vi "Solar Cell Parameters Measuring.vi"() -> ()   [LabVIEW 2019]
uses:
  <vilib>/Analysis/baseanly.llb/Mean (DBL).vi
  <vilib>/DAQmx/create/channels.llb/DAQmx Create Channel (AI-Voltage-Basic).vi
  <vilib>/DAQmx/configure/timing.llb/DAQmx Timing (Sample Clock).vi
  <vilib>/DAQmx/create/channels.llb/DAQmx Create Channel (AO-Voltage-Basic).vi
  <vilib>/DAQmx/miscellaneous.llb/DAQmx Fill In Error Info.vi
  <vilib>/express/express shared/transition.llb/Dynamic To Waveform Array.vi
  <vilib>/express/express signal manip/GetorSetDDTAttributes/Set DDT Attributes/SetT0.vi
  <vilib>/express/express shared/transition.llb/Waveform Array To Dynamic.vi
  <vilib>/express/express signal manip/GetorSetDDTAttributes/Set DDT Attributes/Set DDT Properties.xnode
  <vilib>/DAQmx/read.llb/DAQmx Read (Analog 2D DBL NChan NSamp).vi
  <vilib>/DAQmx/write.llb/DAQmx Write (Analog 1D DBL NChan 1Samp).vi
  <vilib>/DAQmx/read.llb/DAQmx Read (Analog DBL 1Chan 1Samp).vi
  <vilib>/DAQmx/create/channels.llb/DAQmx Create Channel (AI-Temperature-Thermocouple).vi
  <vilib>/Analysis/NI_AALBase.lvlib
  <vilib>/Analysis/NI_AALPro.lvlib
panel:
  in  "Tab Control":enum32{"Parameters", "I-V Curve", "Calibration"}(tab)
  in  "GAIN x":u16(ring)=1000 items=["100"=100, "1000"=1000, "10"=10, "1"=1]
  out "Rseries":dbl format="%#.3g"
  out "Rshunt":dbl format="%#.3g"
  out "Progress":u8(slide)=100 scale=0.0..100.0
  in  "Save File":bool
  in  "S (cm2)":dbl=0.0324
  in  "P  (mW/cm2)":dbl=100.0
  in  "Points":dbl=400.0
  out "Voc  ( V )":dbl format="%#_2g"
  out "Isc  (  mA  )":dbl format="%#_3g"
  out "Imp (mA)":dbl format="%#_3g"
  out "Vmp  (V)":dbl format="%#_2g"
  out "Max  Power  ( mW )":dbl format="%#_2g"
  out "u (%)":dbl format="%#_2g"
  out "FF":dbl format="%#_2g"
  out "Current and Power vs. Voltage":cluster{"voltage":dbl[], "current":dbl[]}[](graph)
  out "Rs":dbl format="%#_3g"
  out "Trmerature Celsius":dbl format="%0.2f"
  in  "File Name":string="Name"
  in  "Grid":enum32{"Radio Selection 1", "Radio Selection 2"}(radio)=enum."Radio Selection 2"
  out "Current (Amps) vs Voltage (Volts)":cluster{"Array":dbl[], "Array":dbl[]}[](graph)
  in  "percentage":sgl=0.075
  in  "100x":dbl=0.00220747 format="%#_13g"
  in  "1000x":dbl=0.01825644 format="%#_13g"
  in  "10x":dbl=0.00069563 format="%#_13g"
  in  "1x":dbl=0.00053122 format="%#_13g"
  out "Gain Coepicient":dbl format="%0.8f"
  out "task out 2":refnum<k21>
  out "task out":refnum<k21>
  # "%"
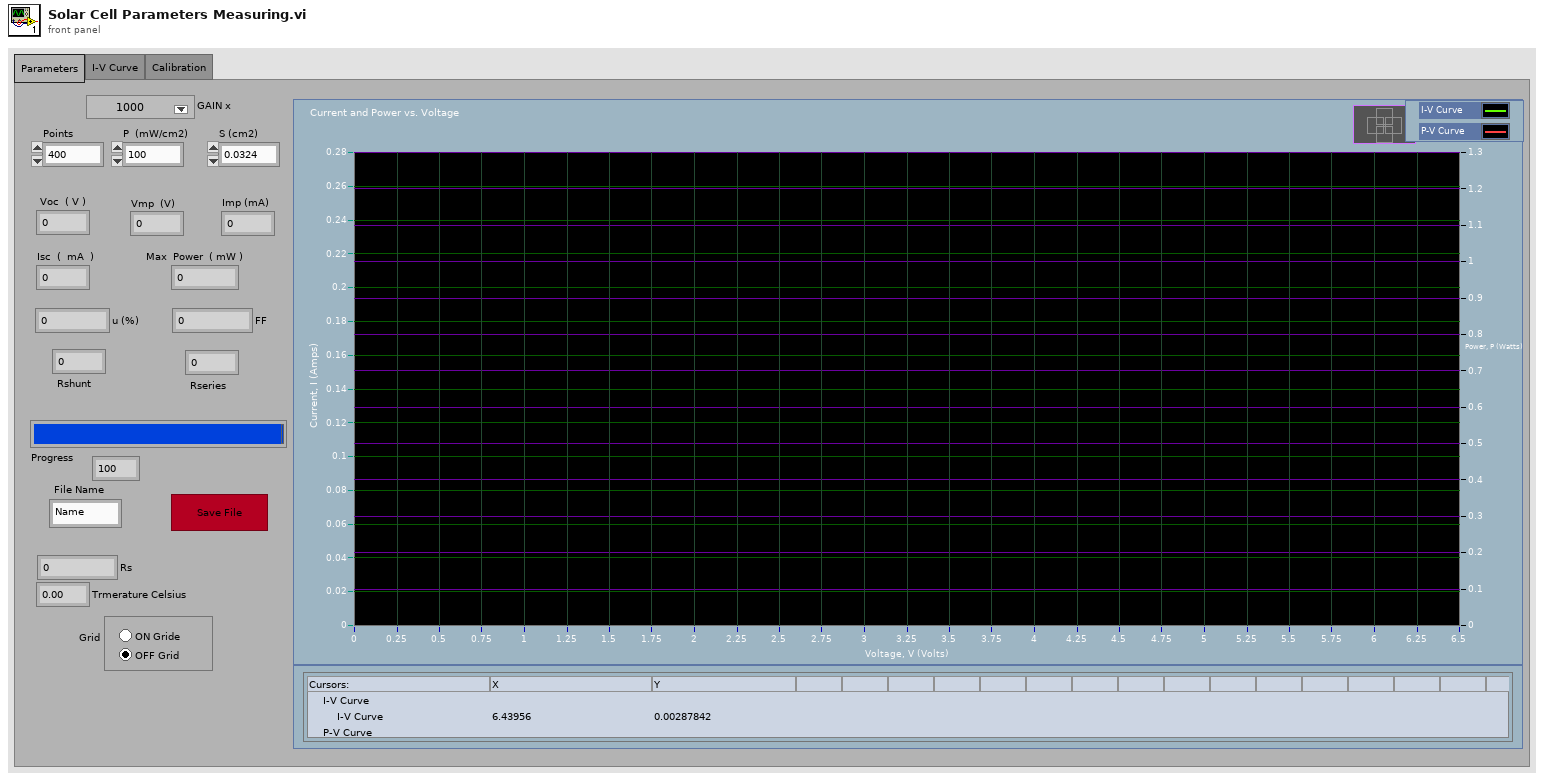
[diagram p1: front panel]
types:
  T1 = typedef "imagedata.ctl" = cluster{"image type":i32, "image depth":i32, "image":u8[], "mask":u8[], "colors":u32[], "Rectangle":cluster{"left":i16, "top":i16, "right":i16, "bottom":i16}}
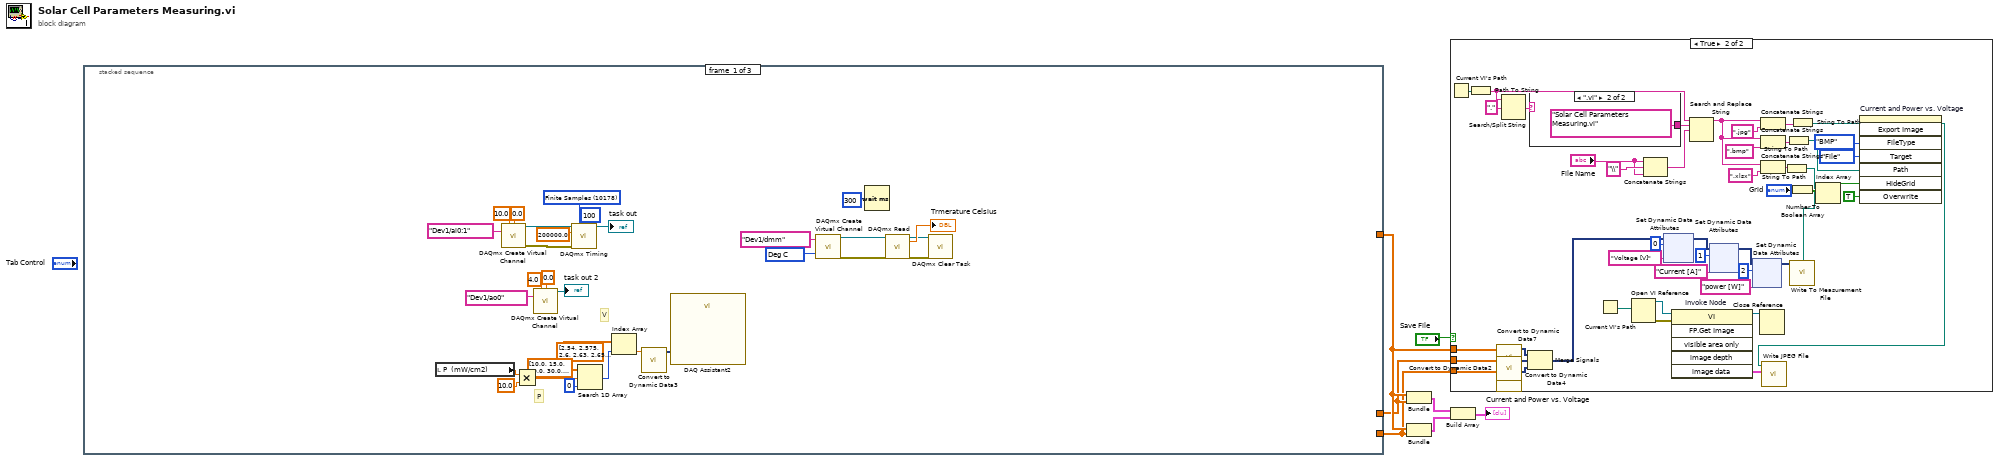
[diagram p0: block diagram]
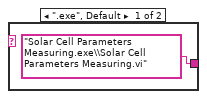
[diagram p3: hidden frame]
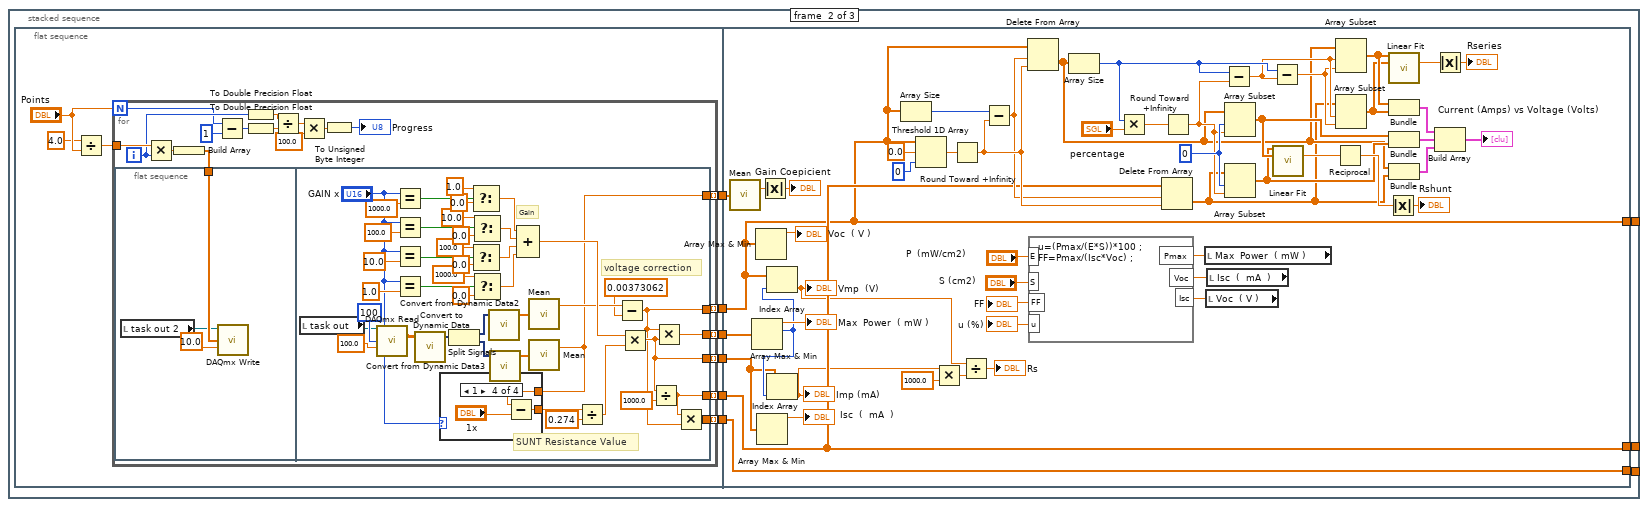
[diagram p4: hidden frame]
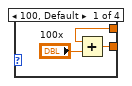
[diagram p5: hidden frame]
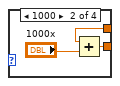
[diagram p6: hidden frame]
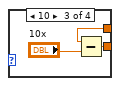
[diagram p7: hidden frame]
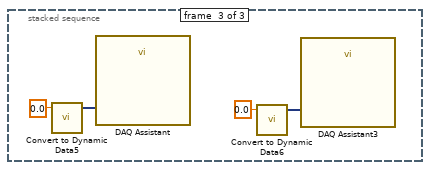
[diagram p8: hidden frame]
diagram:
  n1 = stacked-sequence {
    tunnel: [_ w43 _] -> w3
    tunnel: [_ w40 _] -> w2
    tunnel: [_ w39 _] -> w1
    frame #0 {
      w20 = 10143 items=["Deg C"=10143, "Deg F"=10144, "Kelvins"=10325, "Deg R"=10145, "From Custom Scale"=10065] ("units")
      w26 = 10178 items=["Finite Samples"=10178, "Continuous Samples"=10123, "Hardware Timed Single Point"=12522] ("sample mode")
      # "P"
      # "V"
      n2 = local read "P  (mW/cm2)"() -> (w15:dbl)
      n3 = call-poly <vilib>:"DAQmx Create Virtual Channel.vi"("maximum value"=10.0, "minimum value"=0.0, "physical channels"=tag "Dev1/ai0:1") -> ("task out"=w29:refnum<k21>, "error out"=w28:errorcluster)  [unwired: 11 in]
      n4 = Multiply(x=w15, y=10.0) -> (x*y=w9:dbl)
      n5 = call-poly <vilib>:"DAQmx Create Virtual Channel.vi"("maximum value"=4.0, "minimum value"=0.0, "physical channels"=tag "Dev1/ao0") -> ("task out"=→"task out 2":refnum<k21>)  [unwired: 11 in, 1 out]
      n6 = call-poly <vilib>:"DAQmx Timing.vi"("task/channels in"=w29, "sample mode"=w26, "samples per channel"=100, "rate"=200000.0, "error in"=w28) -> ("task out"=→"task out":refnum<k21>)  [unwired: 9 in, 1 out]
      n7 = Search 1D Array(1D array=dbl[] [10.0, 15.0, 20.0, 30.0, 40.0, 50.0, 60.0, 70.0, 80.0, 90.0, 100.0, 120.0, 140.0, 160.0, 180.0, 200.0, 220.0, 240.0, 260.0, 280.0, 300.0, 350.0, 400.0, 450.0, 500.0, 550.0, 600.0, 650.0, 700.0, 750.0, 800.0, 850.0, 900.0, 950.0, 1000.0] ("P"), element=w9, start index (0)=0) -> (index of element=w10:i32)
      n8 = Index Array(array=dbl[] [2.54, 2.575, 2.6, 2.63, 2.653, 2.672, 2.688, 2.7, 2.71, 2.719, 2.728, 2.74, 2.7525, 2.7627, 2.771, 2.779, 2.784, 2.7895, 2.792, 2.7976, 2.8011, 2.81, 2.817, 2.8238, 2.8295, 2.8301, 2.8315, 2.8325, 2.831, 2.833, 2.835, 2.836, 2.838, 2.84, 2.86] ("V"), index=w10) -> (element=w8:dbl)
      n9 = call "Convert to Dynamic Data3"("Double"=w8) -> ("Dynamic Data Type"=w24:dynamicdata)  [unwired: 3 in]
      n10 = call "DAQ Assistant2"("data"=w24) -> ()  [unwired: 17 in, 2 out]
      n11 = call-poly <vilib>:"DAQmx Create Virtual Channel.vi"("physical channels"=tag "Dev1/dmm", "units"=w20) -> ("task out"=w22:refnum<k21>, "error out"=w19:errorcluster)  [unwired: 12 in]
      n12 = Wait (ms)(milliseconds to wait=u32 300) -> ()  [unwired: 1 out]
      n13 = call-poly <vilib>:"DAQmx Read.vi"("task/channels in"=w22, "error in"=w19) -> ("task out"=w17:refnum<k21>, "data"=→"Trmerature Celsius":dbl, "error out"=w16:errorcluster)  [unwired: 11 in]
      n14 = call <vilib>:"DAQmx Clear Task.vi"("task in"=w17, "error in"=w16) -> ()  [unwired: 13 in, 1 out]
    }
    frame #1 {
      n15 = flat-sequence {
        tunnel: [w52] -> w46
        tunnel: [w51] -> w45
        tunnel: [w50] -> w44
        tunnel: [w49] -> w42
        tunnel: [w48] -> w41
        tunnel: [w47] -> w38
        tunnel: w46 -> [w144]
        tunnel: w45 -> [w136]
        tunnel: w44 -> [w180]
        tunnel: [w144] -> w43
        tunnel: w42 -> [w145]
        tunnel: [w145] -> w40
        tunnel: w41 -> [w142]
        tunnel: [w142] -> w39
        tunnel: w38 -> [w135]
        frame #0 {
          n16 = Divide(x=4.0, y="Points") -> (x/y=w55:dbl)
          n17 = for {
            N: "Points" -> [w62]
            tunnel: w55 -> [w72]
            tunnel: [w61] -> w50 mode=indexing
            tunnel: [w59] -> w52 mode=indexing
            tunnel: [w60] -> w51 mode=indexing
            tunnel: [w58] -> w49 mode=indexing
            tunnel: [w57] -> w48 mode=indexing
            tunnel: [w56] -> w47 mode=indexing
            i -> [w63]
            n18 = flat-sequence {
              tunnel: w74 -> [w77]
              tunnel: [w109] -> w61
              tunnel: [w108] -> w60
              tunnel: [w81] -> w59
              tunnel: [w106] -> w58
              tunnel: [w105] -> w57
              tunnel: [w79] -> w56
              frame #0 {
                n19 = local read "task out 2"() -> (w75:refnum<k21>)
                n20 = call-poly <vilib>:"DAQmx Write.vi"("task/channels in"=w75, "data"=w77, "timeout"=10.0) -> ()  [unwired: 10 in, 3 out]
              }
              frame #1 {
                # "voltage correction"
                # "SUNT Resistance Value"
                # "Gain"
                n21 = local read "task out"() -> (w110:refnum<k21>)
                n22 = call-poly <vilib>:"DAQmx Read.vi"("task/channels in"=w110, "number of samples per channel"=100, "timeout"=100.0) -> ("data"=w115:dbl[][])  [unwired: 10 in, 2 out]
                n23 = Equal?(x="GAIN x", y=1000.0) -> (x = y?=w89:bool)
                n24 = Equal?(x="GAIN x", y=100.0) -> (x = y?=w90:bool)
                n25 = Equal?(x="GAIN x", y=10.0) -> (x = y?=w91:bool)
                n26 = Equal?(x="GAIN x", y=1.0) -> (x = y?=w92:bool)
                n27 = call "Convert to Dynamic Data"("2D Array"=w115) -> ("Dynamic Data Type"=w114:dynamicdata)  [unwired: 3 in]
                n28 = Split Signals(w114) -> (w113:dynamicdata, w112:dynamicdata)  [unwired: 2 in]
                n29 = Select(t=1.0 ("Double"), s=w89, f=0.0) -> (s? t:f=w97:dbl)
                n30 = Select(t=100.0 ("Double"), s=w91, f=0.0) -> (s? t:f=w99:dbl)
                n31 = Select(t=10.0 ("Double"), s=w90, f=0.0) -> (s? t:f=w98:dbl)
                n32 = Select(t=1000.0 ("Double"), s=w92, f=0.0) -> (s? t:f=w100:dbl)
                n33 = call "Convert from Dynamic Data2"("Dynamic Data Type"=w113) -> ("Array"=w118:dbl[])  [unwired: 3 in]
                n34 = call "Convert from Dynamic Data3"("Dynamic Data Type"=w112) -> ("Array"=w119:dbl[])  [unwired: 3 in]
                n35 = Compound Arithmetic op=ADD(w97, w98, w99, w100) -> (w84:dbl)
                n36 = call-poly <vilib>:"Mean.vi"("X"=w118) -> ("mean"=w82:dbl)  [unwired: 1 out]
                n37 = call-poly <vilib>:"Mean.vi"("X"=w119) -> ("mean"=w79:dbl)  [unwired: 1 out]
                n38 = case shown="1" "GAIN x" {
                  tunnel: [w121 w126 w129 w131] -> w78
                  tunnel: w79 -> [w122 w124 w128 w132]
                  frame 100, Default {
                    n39 = Add(x=w122, y="100x") -> (x+y=w121:dbl)
                  }
                  frame 1000 {
                    n40 = Add(x=w124, y="1000x") -> (x+y=w126:dbl)
                  }
                  frame 10 {
                    n41 = Subtract(x=w128, y="10x") -> (x-y=w129:dbl)
                  }
                  frame 1 {
                    n42 = Subtract(x=w132, y="1x") -> (x-y=w131:dbl)
                  }
                }
                n43 = Divide(x=w78, y=0.274) -> (x/y=w116:dbl)
                n44 = Subtract(x=w82, y=0.00373062) -> (x-y=w81:dbl)
                n45 = Multiply(x=w84, y=w116) -> (x*y=w108:dbl)
                n46 = Divide(x=w108, y=1000.0) -> (x/y=w106:dbl)
                n47 = Multiply(x=w81, y=w108) -> (x*y=w109:dbl)
                n48 = Multiply(x=w106, y=w81) -> (x*y=w105:dbl)
              }
            }
            n49 = Multiply(x=w72, y=w63) -> (x*y=w73:dbl)
            n50 = Build Array(w73) -> (w74:dbl[])
            n51 = Subtract(x=w62, y=1) -> (x-y=w65:i32)
            n52 = To Double Precision Float(number=w63) -> (double precision float=w66:dbl)
            n53 = To Double Precision Float(number=w65) -> (double precision float=w68:dbl)
            n54 = Divide(x=w66, y=w68) -> (x/y=w70:dbl)
            n55 = Multiply(x=w70, y=100.0) -> (x*y=w67:dbl)
            n56 = To Unsigned Byte Integer(number=w67) -> (unsigned 8bit integer=→"Progress":u8)
          }
        }
        frame #1 {
          w158 = 0 ("index")
          n57 = call-poly <vilib>:"Mean.vi"("X"=w135) -> ("mean"=w134:dbl)  [unwired: 1 out]
          n58 = Array Max & Min(array=w180) -> (max value=→"Max  Power  ( mW )":dbl, max index (indices)=w181:i32)  [unwired: 2 out]
          n59 = Array Max & Min(array=w144) -> (max value=→"Voc  ( V )":dbl)  [unwired: 3 out]
          n60 = Array Max & Min(array=w136) -> (max value=→"Isc  (  mA  )":dbl)  [unwired: 3 out]
          n61 = Absolute Value(x=w134) -> (abs(x)=→"Gain Coepicient":dbl)
          n62 = Index Array(array=w144, index=w181) -> (element=w137:dbl)
          "Vmp  (V)" <- w137
          n63 = Index Array(array=w136, index=w181) -> (element=w139:dbl)
          "Imp (mA)" <- w139
          n64 = Array Size(array=w144) -> (size(s)=w157:i32)
          n65 = Threshold 1D Array(1:0 ("start index (0)"), 2:0.0 ("threshold y"), 3:w144) -> (0:w170:dbl)
          n66 = Multiply(x=w139, y=1000.0) -> (x*y=w140:dbl)
          n67 = Round Toward +Infinity(x=w170) -> (ceil(x): smallest int >= x=w169:dbl)
          n68 = Divide(x=w137, y=w140) -> (x/y=→"Rs":dbl)
          n69 = Subtract(x=w157, y=w169) -> (x-y=w168:dbl)
          n70 = Delete From Array(array=w144, length=w168, index=w169) -> (deleted portion=w152:dbl[])  [unwired: 1 out]
          n71 = Array Size(array=w152) -> (size(s)=w155:i32)
          n72 = Multiply(x=w155, y="percentage") -> (x*y=w163:sgl)
          n73 = Delete From Array(array=w145, length=w168, index=w169) -> (deleted portion=w151:dbl[])  [unwired: 1 out]
          n74 = Round Toward +Infinity(x=w163) -> (ceil(x): smallest int >= x=w156:sgl)
          n75 = local read "Max  Power  ( mW )"() -> (w177:dbl)
          n76 = local read "Voc  ( V )"() -> (w179:dbl)
          n77 = local read "Isc  (  mA  )"() -> (w178:dbl)
          n78 = formula code="u=(Pmax/(E*S))*100 ;\nFF=Pmax/(Isc*Voc) ;"("Voc"=w178, "Isc"=w179, "E"="P  (mW/cm2)", "S"="S (cm2)", "Pmax"=w177) -> ("FF"=→"FF":dbl, "u"=→"u (%)":dbl)
          n79 = Subtract(x=w155, y=w156) -> (x-y=w154:sgl)
          n80 = Array Subset(array=w152, index=w158, length=w156) -> (w162:dbl[])
          n81 = Array Subset(array=w151, index=w158, length=w156) -> (w161:dbl[])
          n82 = Subtract(x=w155, y=w154) -> (x-y=w153:sgl)
          n83 = call <vilib>:"Linear Fit.vi"("Y"=w161, "X"=w162) -> ("slope"=w167:dbl)  [unwired: 4 in, 9 out]
          n84 = Reciprocal(x=w167) -> (1/x=w166:dbl)
          n85 = Array Subset(array=w152, index=w154, length=w153) -> (w149:dbl[])
          n86 = Array Subset(array=w151, index=w154, length=w153) -> (w148:dbl[])
          n87 = Absolute Value(x=w166) -> (abs(x)=→"Rshunt":dbl)
          n88 = call <vilib>:"Linear Fit.vi"("Y"=w149, "X"=w148) -> ("slope"=w147:dbl)  [unwired: 4 in, 9 out]
          n89 = Bundle(w149, w148) -> (w146:cluster{dbl[], dbl[]})  [unwired: 1 out]
          n90 = Bundle(w162, w161) -> (w159:cluster{dbl[], dbl[]})  [unwired: 1 out]
          n91 = Bundle(w152, w151) -> (w160:cluster{dbl[], dbl[]})  [unwired: 1 out]
          n92 = Absolute Value(x=w147) -> (abs(x)=→"Rseries":dbl)
          n93 = Build Array(w146, w159, w160) -> (→"Current (Amps) vs Voltage (Volts)":cluster{dbl[], dbl[]}[])
        }
      }
    }
    frame #2 {
      n94 = call "Convert to Dynamic Data5"("Double"=0.0) -> ("Dynamic Data Type"=w187:dynamicdata)  [unwired: 3 in]
      n95 = call "DAQ Assistant"("data"=w187) -> ()  [unwired: 17 in, 2 out]
      n96 = call "Convert to Dynamic Data6"("Double"=0.0) -> ("Dynamic Data Type"=w185:dynamicdata)  [unwired: 3 in]
      n97 = call "DAQ Assistant3"("data"=w185) -> ()  [unwired: 17 in, 2 out]
    }
  }
  n98 = Bundle(w3, w2) -> (w6:cluster{dbl[], dbl[]})  [unwired: 1 in]
  n99 = Bundle(w3, w1) -> (w5:cluster{dbl[], dbl[]})  [unwired: 1 in]
  n100 = case shown="True" "Save File" {
    tunnel: w2 -> [_ w233]
    tunnel: w1 -> [_ w232]
    tunnel: w3 -> [_ w218]
    frame False {
    }
    frame True {
      n101 = Current VI's Path() -> (path=w201:path)
      n102 = Path To String(path=w201) -> (string=w202:string)
      n103 = call "Convert to Dynamic Data7"("Array"=w218) -> ("Dynamic Data Type"=w214:dynamicdata)  [unwired: 3 in]
      n104 = call "Convert to Dynamic Data2"("Array"=w233) -> ("Dynamic Data Type"=w215:dynamicdata)  [unwired: 3 in]
      n105 = call "Convert to Dynamic Data4"("Array"=w232) -> ("Dynamic Data Type"=w216:dynamicdata)  [unwired: 3 in]
      n106 = Search/Split String(string=w202, search string/char (-)=".") -> (match + rest of string=w200:string)  [unwired: 1 in, 2 out]
      n107 = Merge Signals(w214, w215, w216) -> (w213:dynamicdata)
      n108 = case shown="\".vi\"" w200 {
        tunnel: ["Solar Cell Parameters Measuring.exe\\Solar Cell Parameters Measuring.vi" ("regular expression") "Solar Cell Parameters Measuring.vi" ("regular expression")] -> w199
        frame ".exe", Default {
        }
        frame ".vi" {
        }
      }
      n109 = Current VI's Path() -> (path=w227:path)
      n110 = Open VI Reference(vi path=w227) -> (vi reference=w228:refnum<vi>, error out=w229:errorcluster)  [unwired: 5 in]
      n111 = Concatenate Strings("File Name", "\\" ("string"), "File Name") -> (w192:string)
      n112 = xnode ("Set Dynamic Data Attributes")("Signals In"=w213, "Signal Index"=0, "Signal Name"="Voltage [V]") -> ("Signals Out"=w226:dynamicdata)  [unwired: 1 in, 1 out]
      n113 = invoke on="Invoke Node" class="VI" method="FP.Get Image"(reference=w228, error in=w229) -> (reference out=w231:refnum<vi>, "image data"=w230:T1)  [unwired: 4 in, 4 out]
      n114 = Search and Replace String(input string=w202, search string=w199, replace string=w192) -> (result string=w195:string)  [unwired: 5 in, 3 out]
      n115 = xnode ("Set Dynamic Data Attributes")("Signals In"=w226, "Signal Index"=1, "Signal Name"="Current [A]") -> ("Signals Out"=w219:dynamicdata)  [unwired: 1 in, 1 out]
      n116 = xnode ("Set Dynamic Data Attributes")("Signals In"=w219, "Signal Index"=2, "Signal Name"="power [W]") -> ("Signals Out"=w217:dynamicdata)  [unwired: 1 in, 1 out]
      n117 = Close Reference(reference=w231) -> ()  [unwired: 1 in, 1 out]
      n118 = Concatenate Strings(w195, ".jpg" ("string")) -> (w197:string)
      n119 = Concatenate Strings(w195, ".bmp" ("string")) -> (w190:string)
      n120 = Concatenate Strings(w195, ".xlsx" ("string")) -> (w189:string)
      n121 = String To Path(string=w189) -> (path=w210:path)
      n122 = String To Path(string=w190) -> (path=w204:path)
      n123 = call "Write To Measurement File"("Signals"=w217, "Filename"=w210) -> ()  [unwired: 15 in, 3 out]
      n124 = String To Path(string=w197) -> (path=w209:path)
      n125 = call <vilib>:"Write JPEG File.vi"("image data"=w230, "path to JPEG file"=w209) -> ()  [unwired: 8 in, 2 out]
      n126 = Number To Boolean Array(number="Grid") -> (Boolean array=w211:bool[])
      n127 = Index Array(array=w211) -> (element=w208:bool)  [unwired: 1 in]
      n128 = invoke on="Current and Power vs. Voltage" class="XYGraph (strict)" method="Export Image"("FileType"=enum32{"BMP", "EPS", "EMF", "PICT"}."BMP" ("File Type"), "Target"=enum32{"File", "Clipboard"}."File", "Path"=w204, "HideGrid"=w208, "Overwrite"=TRUE ("Always Overwrite")) -> ()  [unwired: 3 in, 8 out]
    }
  }
  n129 = Build Array(w6, w5) -> (→"Current and Power vs. Voltage":cluster{dbl[], dbl[]}[])
